vi "Read As Stream_Cancel.vi"(8 "error in (no error)":errorcluster, 11 "HttpContent in":refnum<class "HttpContent.lvclass">) -> (0 "error out":errorcluster, 3 "HttpContent out":refnum<class "HttpContent.lvclass">)   [LabVIEW 2018, in "LabVIEWHTTPClient_NET.lvlib" / "HttpContent.lvclass"]
uses:
  HttpContent.lvclass
  HttpContent.lvclass/HttpContent.ctl
  Accessors/Read NET_StreamCancellationSource.vi
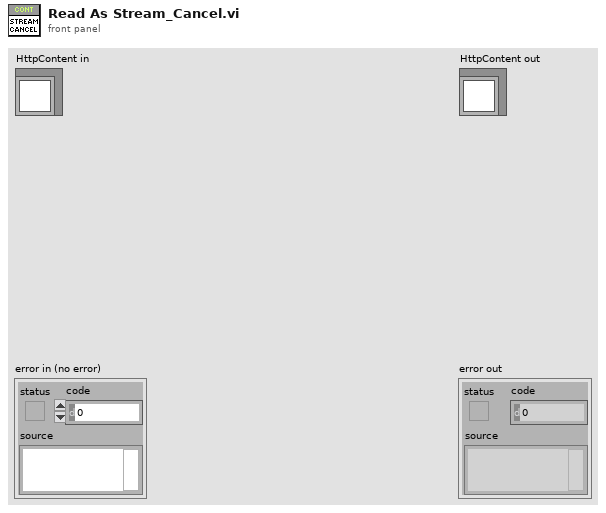
[diagram p1: front panel]
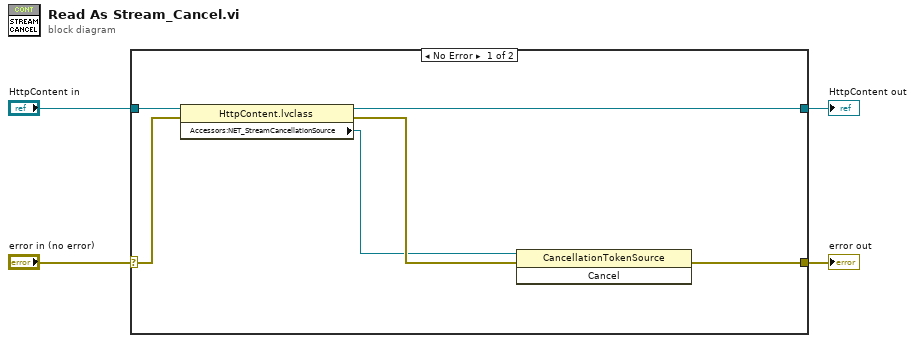
[diagram p0: block diagram]
diagram:
  n1 = case shown="No Error" "error in (no error)" {
    selector: "error in (no error)" -> [w10 w12]
    tunnel: [w6 w12] -> w3
    tunnel: [w7 w11] -> w1
    tunnel: "HttpContent in" -> [w8 w11]
    frame No Error {
      n2 = property class="HttpContent.lvclass"(reference=w8, error in=w10) -> (reference out=w7:refnum<class "HttpContent.lvclass">, error out=w9:errorcluster, "Accessors:NET_StreamCancellationSource"=w5:refnum<k24>)
      n3 = invoke class="CancellationTokenSource" method="Cancel"(reference=w5, error in=w9) -> (error out=w6:errorcluster)  [unwired: 1 in, 2 out]
    }
    frame Error {
    }
  }
  "error out" <- w3
  "HttpContent out" <- w1
